vi "GetNodePort.vi"(1 "ROS in":T1={"topic port"=0, "Node"="", "topic"="", "type"="", "node port"=0, "error "={"status"=FALSE, "code"=0, "source"=""}, "Direction"=enum."Node", "APIs"=[], "Update (ms)"=1, "write queue"=1}) -> (0 "ROS out":T1={"topic port"=0, "Node"="", "topic"="", "type"="", "node port"=0, "error "={"status"=FALSE, "code"=0, "source"=""}, "Direction"=enum."Node", "APIs"=[], "Update (ms)"=1, "write queue"=1})   [LabVIEW 2012]
uses:
  <userlib>/ROSforLV/ROS/Code/SubVIs/_ROSControl.ctl
  <userlib>/ROSforLV/ROS/Code/SubVIs/_ROSDirection.ctl
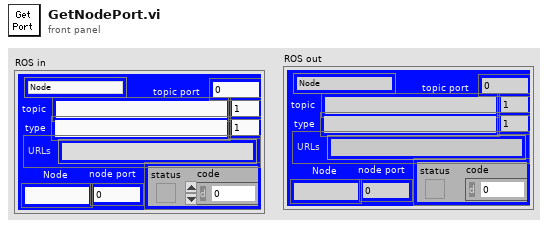
[diagram p1: front panel]
types:
  T1 = typedef "_ROSControl.ctl" = cluster{"topic port":u16, "Node":string, "topic":string, "type":string, "node port":u16, "error ":errorcluster, "Direction":T2, "APIs":string[], "Update (ms)":u16, "write queue":u16}
  T2 = typedef "_ROSDirection.ctl" = enum16{"Node", "Publisher", "Subscriber", "Service Client"}
  T3 = typedef "ServoInfo.ctl" = cluster{"vi name":string, "VI Refnum":refnum<vi>, "queue":refnum<queue>, "ROS":T1, "notifier":refnum<notifier>}
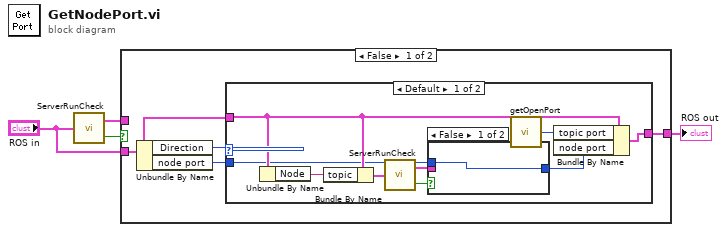
[diagram p0: block diagram]
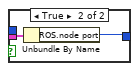
[diagram p2: hidden frame]
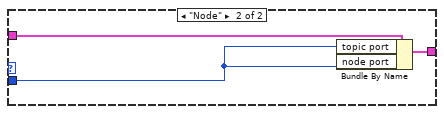
[diagram p3: hidden frame]
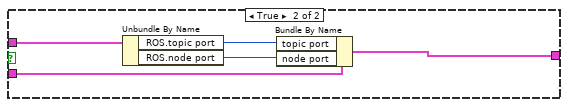
[diagram p4: hidden frame]
diagram:
  n1 = call <userlib>:"ServerRunCheck.vi"("ROS in"="ROS in") -> ("Running?"=w4:bool, "ServerFound"=w1:T3)
  n2 = case shown="False" w4 {
    tunnel: "ROS in" -> [w6 w27]
    tunnel: [w7 w24] -> w2
    tunnel: w1 -> [_ w28]
    frame False {
      n3 = Unbundle By Name(w6) -> ("Direction"=w8:T2, "node port"=w5:u16)
      n4 = case shown="Default" w8 {
        tunnel: w6 -> [w13 w23]
        tunnel: [w16 w22] -> w7
        tunnel: w5 -> [w9 w21]
        frame Default {
          n5 = Unbundle By Name(w13) -> ("Node"=w15:string)
          n6 = Bundle By Name(cluster=w13, "topic"=w15) -> (w12:T1)
          n7 = call <userlib>:"ServerRunCheck.vi"("ROS in"=w12) -> ("Running?"=w10:bool, "ServerFound"=w14:T3)
          n8 = case shown="False" w10 {
            tunnel: w14 -> [_ w20]
            tunnel: [w18 w19] -> w11
            tunnel: w9 -> [w18 _]
            frame False {
            }
            frame True {
              n9 = Unbundle By Name(w20) -> ("ROS.node port"=w19:u16)
            }
          }
          n10 = call <userlib>:"getOpenPort.vi"() -> ("port"=w17:u16)
          n11 = Bundle By Name(cluster=w13, "topic port"=w17, "node port"=w11) -> (w16:T1)
        }
        frame "Node" {
          n12 = Bundle By Name(cluster=w23, "topic port"=w21, "node port"=w21) -> (w22:T1)
        }
      }
    }
    frame True {
      n13 = Unbundle By Name(w28) -> ("ROS.topic port"=w26:u16, "ROS.node port"=w25:u16)
      n14 = Bundle By Name(cluster=w27, "topic port"=w26, "node port"=w25) -> (w24:T1)
    }
  }
  "ROS out" <- w2
